vi "Agua_llenado_02.vi"() -> ()   [LabVIEW 2022 SP3]
uses:
  <vilib>/Instr/_visa.llb/VISA Configure Serial Port (Instr).vi
panel:
  in  "Habilitado":bool
  in  "VISA resource name":refnum<visa-resource-name>
  in  "ms/Ciclo":dbl=50.0
  out "mLs":dbl
  out "Llenando...":bool
  out "Listo":bool=TRUE
  in  "500 ml":bool
  in  "250 ml":bool
  out "Vasito":dbl(slide) scale=0.0..500.0
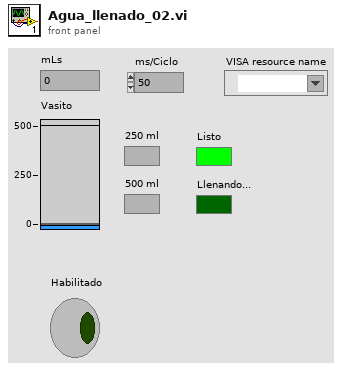
[diagram p1: front panel]
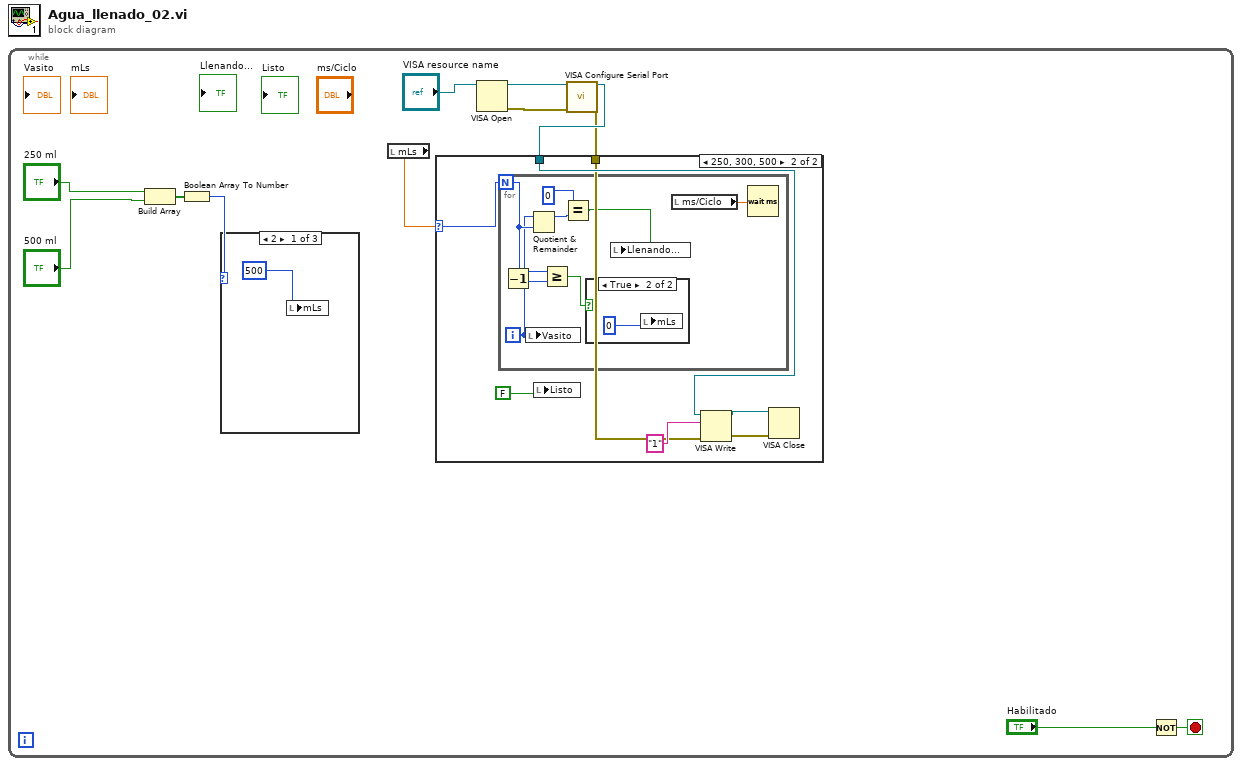
[diagram p0: block diagram]
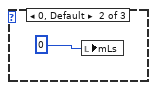
[diagram p2: hidden frame]
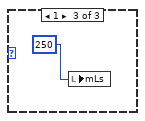
[diagram p3: hidden frame]
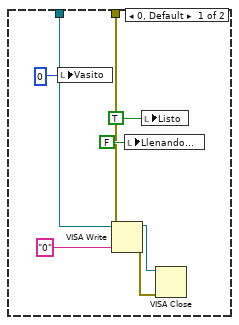
[diagram p4: hidden frame]
diagram:
  n1 = while {
    stop <- w8 stop-if-true
    n2 = Build Array("250 ml", "500 ml") -> (w12:bool[])
    n3 = Boolean Array To Number(Boolean array=w12) -> (number=w9:u32)
    n4 = case shown="2" w9 {
      frame 2 {
        n5 = local write "mLs"(500) -> ()
      }
      frame 0, Default {
        n6 = local write "mLs"(0) -> ()
      }
      frame 1 {
        n7 = local write "mLs"(250) -> ()
      }
    }
    n8 = local read "mLs"() -> (w7:dbl)
    n9 = VISA Open(VISA resource name="VISA resource name") -> (VISA resource name=w5:refnum<visa-resource-name>, error out=w4:errorcluster)  [unwired: 4 in]
    n10 = call-poly "VISA Configure Serial Port"("VISA resource name"=w5, "error in (no error)"=w4) -> ("VISA resource name out"=w3:refnum<visa-resource-name>, "error out"=w2:errorcluster)  [unwired: 12 in]
    n11 = case shown="250, 300, 500" w7 {
      selector: w7 -> [_ w29]
      tunnel: w3 -> [w19 w27]
      tunnel: w2 -> [w18 w26]
      frame 0, Default {
        n12 = local write "Vasito"(0) -> ()
        n13 = VISA Write(VISA resource name=w19, write buffer="0", error in (no error)=w18) -> (VISA resource name out=w17:refnum<visa-resource-name>, error out=w16:errorcluster)  [unwired: 1 out]
        n14 = local write "Llenando..."(FALSE) -> ()
        n15 = local write "Listo"(TRUE) -> ()
        n16 = VISA Close(VISA resource name=w17, error in (no error)=w16) -> ()  [unwired: 1 out]
      }
      frame 250, 300, 500 {
        n17 = for {
          N: w29 -> [w33]
          i -> [w32]
          n18 = Decrement(x=w33) -> (x-1=w36:i32)
          n19 = local write "Vasito"(w32) -> ()
          n20 = Quotient & Remainder(x=w32, y=w33) -> (x-y*floor(x/y)=w34:i32)  [unwired: 1 out]
          n21 = Greater Or Equal?(x=w32, y=w36) -> (x >= y?=w35:bool)
          n22 = Equal?(x=0, y=w34) -> (x = y?=w38:bool)
          n23 = case shown="True" w35 {
            frame False {
            }
            frame True {
              n24 = local write "mLs"(0) -> ()
            }
          }
          n25 = local write "Llenando..."(w38) -> ()
          n26 = local read "ms/Ciclo"() -> (w31:dbl)
          n27 = Wait (ms)(milliseconds to wait=w31) -> ()  [unwired: 1 out]
        }
        n28 = local write "Listo"(FALSE) -> ()
        n29 = VISA Write(VISA resource name=w27, write buffer="1", error in (no error)=w26) -> (VISA resource name out=w25:refnum<visa-resource-name>, error out=w24:errorcluster)  [unwired: 1 out]
        n30 = VISA Close(VISA resource name=w25, error in (no error)=w24) -> ()  [unwired: 1 out]
      }
    }
    n31 = Not(x="Habilitado") -> (.not. x?=w8:bool)
  }
